vi "RF_Attn_commands.vi"(1 "Value":dbl, 2 "Insertion Loss":dbl, 3 "Parameter":enum16{"Attenuation (dB)"}(ring)) -> (0 "Command (dB)":dbl)   [LabVIEW 2013]
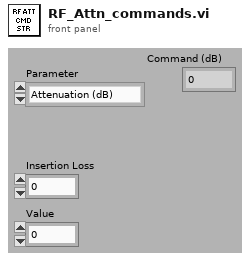
[diagram p1: front panel]
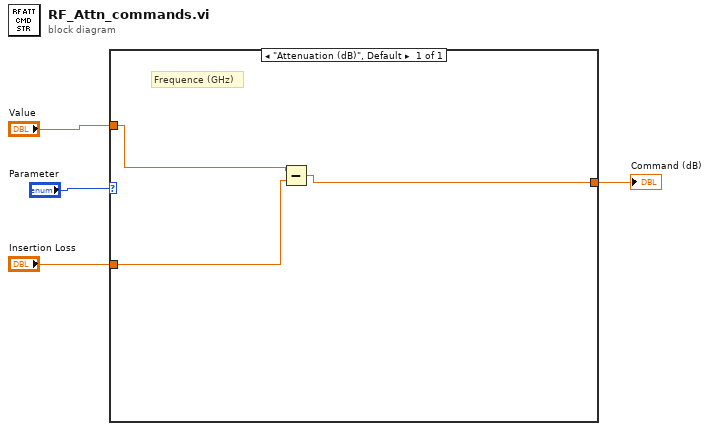
[diagram p0: block diagram]
diagram:
  n1 = case shown="\"Attenuation (dB)\", Default" "Parameter" {
    tunnel: "Value" -> [w7]
    tunnel: [w5] -> w1
    tunnel: "Insertion Loss" -> [w6]
    frame "Attenuation (dB)", Default {
      # "Frequence (GHz)"
      n2 = Subtract(x=w7, y=w6) -> (x-y=w5:dbl)
    }
  }
  "Command (dB)" <- w1
